vi "Created Attributes.vi"(10 "Alias":string, 11 "Base Actor in":refnum<class "Base Actor.lvclass">) -> (1 "Is Found":bool, 2 "Created Attributes":T1)   [LabVIEW 2020, in "jettl.lvlib" / "Actor.lvlib" / "Base Actor.lvclass"]
uses:
  Base Actor.lvclass
  Msg/Msg.lvclass
  Implemented Msgs.ctl
  Actor.lvlib
  Attributes.ctl
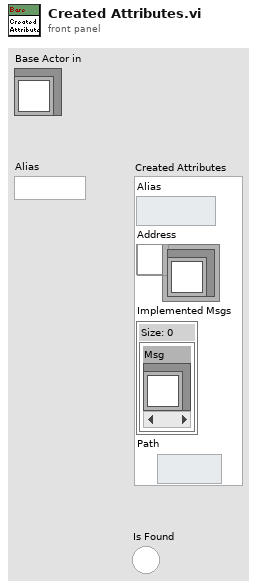
[diagram p1: front panel]
types:
  T1 = typedef "jettl.lvlib/Actor.lvlib/Attributes.ctl" = cluster{"Alias":string, "Address":refnum<user-event>, "Implemented Msgs":T2, "Path":path}
  T2 = typedef "jettl.lvlib/Actor.lvlib/Implemented Msgs.ctl" = set{refnum<class "Msg.lvclass">}
  T3 = typedef "jettl.lvlib/Actor.lvlib/Alias to Created Attributes.ctl" = map{string, T1}
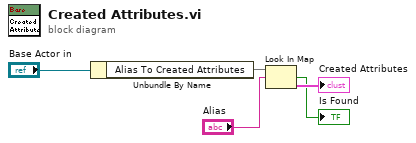
[diagram p0: block diagram]
diagram:
  n1 = Unbundle By Name("Base Actor in") -> ("Alias To Created Attributes"=w4:T3)
  n2 = Look In Map(map=w4, key="Alias") -> (key not found?=→"Is Found":bool, value=→"Created Attributes":T1)  [unwired: 1 in]
